vi "Init UI Elements.vi"(6 "Valid SDF?":bool, 7 "This VI":refnum<vi>, 8 "error in (no error)":errorcluster, 11 "Loop Data in":T1) -> (0 "error out":errorcluster, 3 "Loop Data out":T1)   [LabVIEW 2016, in "System Mapping Tool.lvlib"]
uses:
  System Mapping Tool.lvlib
  TypeDefs/Loop Data.ctl
  TypeDefs/UI Refs.ctl
  NationalInstruments.VeriStand.SystemDefinitionAPI
  NationalInstruments.VeriStand.SystemStorageUI
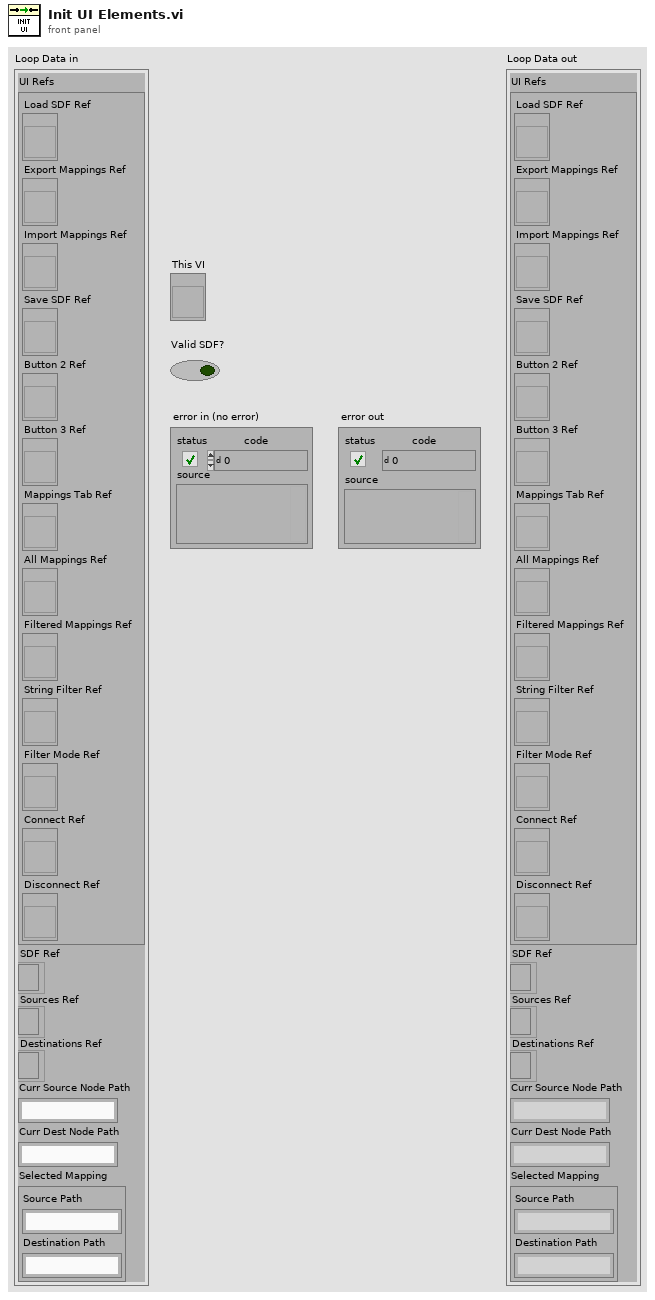
[diagram p1: front panel]
types:
  T1 = typedef "System Mapping Tool.lvlib/Loop Data.ctl" = cluster{"UI Refs":T2, "SDF Ref":refnum<k24>, "Sources Ref":refnum<k24>, "Destinations Ref":refnum<k24>, "Curr Source Node Path":string, "Curr Dest Node Path":string, "Selected Mapping":cluster{"Source Path":string, "Destination Path":string}}
  T2 = typedef "System Mapping Tool.lvlib/UI Refs.ctl" = cluster{"Load SDF Ref":refnum<vi>, "Export Mappings Ref":refnum<vi>, "Import Mappings Ref":refnum<vi>, "Save SDF Ref":refnum<vi>, "Button 2 Ref":refnum<vi>, "Button 3 Ref":refnum<vi>, "Mappings Tab Ref":refnum<vi>, "All Mappings Ref":refnum<vi>, "Filtered Mappings Ref":refnum<vi>, "String Filter Ref":refnum<vi>, "Filter Mode Ref":refnum<vi>, "Connect Ref":refnum<vi>, "Disconnect Ref":refnum<vi>}
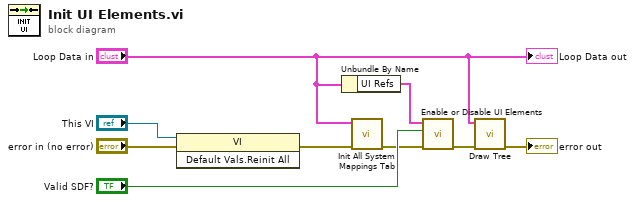
[diagram p0: block diagram]
diagram:
  n1 = invoke class="VI" method="Default Vals.Reinit All"(reference="This VI", error in="error in (no error)") -> (error out=w6:errorcluster)  [unwired: 1 in, 2 out]
  n2 = Unbundle By Name("Loop Data in") -> ("UI Refs"=w4:T2)
  n3 = call "Init All System Mappings Tab.vi"("error in (no error)"=w6, "Loop Data in"="Loop Data in") -> ("error out"=w5:errorcluster)  [unwired: 9 in]
  n4 = call "Enable or Disable UI Elements.vi"("error in (no error)"=w5, "Enable?"="Valid SDF?", "UI Refs in"=w4) -> ("error out"=w3:errorcluster)  [unwired: 7 in, 1 out]
  n5 = call "Draw Tree.vi"("error in (no error)"=w3, "Loop Data"="Loop Data in") -> ("error out"=→"error out":errorcluster)  [unwired: 9 in]
  "Loop Data out" <- "Loop Data in"
